vi "Endpoint String.vi"(4 "Port":u16, 5 "Address":string) -> (1 "Endpoint":string)   [LabVIEW 2020, in "Volatus.lvlib"]
uses:
  Volatus.lvlib
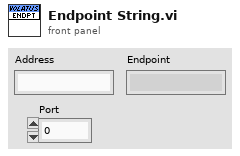
[diagram p1: front panel]
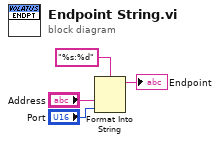
[diagram p0: block diagram]
diagram:
  n1 = Format Into String(format string="%s:%d", "Address", "Port") -> (resulting string=→"Endpoint":string)  [unwired: 2 in, 1 out]
